vi "Translator.File.MatchStrings (Array).vi"(4 "sort? (T)":bool=TRUE, 5 "progressbar":refnum<vi>, 7 "group":string, 8 "error in":errorcluster, 9 "labels":string[](array[string]), 10 "default values":string[](array[string]), 11 "refnum in":T1) -> (0 "error out":errorcluster, 1 "#added":i32, 2 "values out":string[](array[string]), 3 "refnum out":T1)   [LabVIEW 2016]
uses:
  <vilib>/Utility/config.llb/Config Data RefNum.ctl
  <vilib>/Utility/config.llb/Write Key (String).vi
  <vilib>/Utility/config.llb/Read Key (String).vi
  <vilib>/Utility/config.llb/NI_LVConfig.lvlib
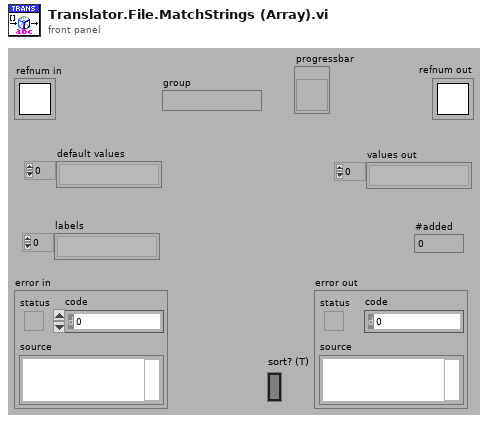
[diagram p1: front panel]
types:
  T1 = typedef "NI_LVConfig.lvlib/Config Data RefNum.ctl" = refnum<k1>
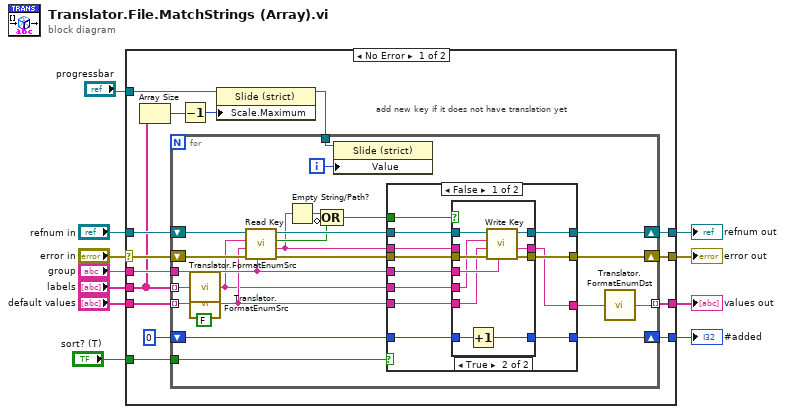
[diagram p0: block diagram]
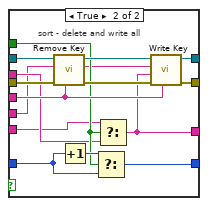
[diagram p3: hidden frame]
diagram:
  n1 = case shown="No Error" "error in" {
    selector: "error in" -> [w19 w91]
    tunnel: "refnum in" -> [w18 w92]
    tunnel: [w25 _] -> w10
    tunnel: [w24 w92] -> w9
    tunnel: [w23 w91] -> w8
    tunnel: [w22 w90] -> w7
    tunnel: "group" -> [w21 _]
    tunnel: "labels" -> [w15 _]
    tunnel: "default values" -> [w20 w90]
    tunnel: "progressbar" -> [w14 _]
    tunnel: "sort? (T)" -> [w12 _]
    frame No Error {
      # "add new key if it does not have translation yet"
      n2 = Array Size(array=w15) -> (size(s)=w17:i32)
      n3 = Decrement(x=w17) -> (x-1=w16:i32)
      n4 = property on="Property Node" class="Slide (strict)"(reference=w14, "Scale.Maximum"=w16) -> (reference out=w13:refnum<vi>)  [unwired: 1 in, 1 out]
      n5 = for {
        tunnel: w21 -> [w43]
        tunnel: w15 -> [w42] mode=indexing
        shift-right: [w46] -> w23
        shift-left: w19 -> [w49]
        shift-right: [w44] -> w24
        shift-left: w18 -> [w48]
        tunnel: [w28] -> w22 mode=indexing
        shift-right: [w34] -> w25
        shift-left: 0 -> [w35]
        tunnel: w20 -> [w41] mode=indexing
        tunnel: w13 -> [w32]
        tunnel: w12 -> [w29]
        i -> [w30]
        n6 = call "Translator.FormatEnumSrc.vi"("text in"=w42) -> ("text out"=w31:string)  [unwired: 1 in]
        n7 = call "Translator.FormatEnumSrc.vi"("text in"=w41, "quotas?(T)"=FALSE) -> ("text out"=w40:string)
        n8 = call-poly <vilib>:"Read Key.vi"("section"=w43, "error in (no error)"=w49, "default value"=w40, "key"=w31, "refnum"=w48) -> ("error out"=w47:errorcluster, "value"=w36:string, "found?"=w37:bool, "refnum out"=w45:T1)  [unwired: 3 in]
        n9 = Empty String/Path?(string/path=w36) -> (empty?=w39:bool)
        n10 = Compound Arithmetic op=OR(w39, invert w37) -> (w38:bool)
        n11 = property on="Property Node" class="Slide (strict)"(reference=w32, "Value"=w30) -> ()  [unwired: 1 in, 2 out]
        n12 = case shown="False" w29 {
          tunnel: w47 -> [w61 w89]
          tunnel: [w60 w84] -> w46
          tunnel: w45 -> [w59 w88]
          tunnel: [w58 w86] -> w44
          tunnel: w43 -> [w57 w83]
          tunnel: w40 -> [w56 w77]
          tunnel: w38 -> [w55 w79]
          tunnel: w36 -> [w54 w78]
          tunnel: w35 -> [w53 w82]
          tunnel: [w52 w80] -> w34
          tunnel: w31 -> [w51 w75]
          tunnel: [w50 w76] -> w27
          frame False {
            n13 = case shown="True" w55 {
              tunnel: w61 -> [w64 w74]
              tunnel: [w64 w73] -> w60
              tunnel: w59 -> [w65 w72]
              tunnel: [w65 w71] -> w58
              tunnel: w57 -> [_ w70]
              tunnel: w56 -> [_ w66]
              tunnel: w54 -> [w63 _]
              tunnel: w51 -> [_ w69]
              tunnel: [w63 w66] -> w50
              tunnel: w53 -> [w62 w68]
              tunnel: [w62 w67] -> w52
              frame False {
              }
              frame True {
                n14 = Increment(x=w68) -> (x+1=w67:i32)
                n15 = call-poly <vilib>:"Write Key.vi"("section"=w70, "error in (no error)"=w74, "value"=w66, "key"=w69, "refnum"=w72) -> ("error out"=w73:errorcluster, "refnum out"=w71:T1)  [unwired: 4 in, 1 out]
              }
            }
          }
          frame True {
            # "sort - delete and write all"
            n16 = call <vilib>:"Remove Key.vi"("section"=w83, "error in (no error)"=w89, "key"=w75, "refnum"=w88) -> ("error out"=w85:errorcluster, "refnum out"=w87:T1)  [unwired: 5 in, 1 out]
            n17 = Increment(x=w82) -> (x+1=w81:i32)
            n18 = Select(t=w81, s=w79, f=w82) -> (s? t:f=w80:i32)
            n19 = Select(t=w77, s=w79, f=w78) -> (s? t:f=w76:string)
            n20 = call-poly <vilib>:"Write Key.vi"("section"=w83, "error in (no error)"=w85, "value"=w76, "key"=w75, "refnum"=w87) -> ("error out"=w84:errorcluster, "refnum out"=w86:T1)  [unwired: 4 in, 1 out]
          }
        }
        n21 = call "Translator.FormatEnumDst.vi"("text in"=w27) -> ("text out"=w28:string)
      }
    }
    frame Error {
    }
  }
  "#added" <- w10
  "refnum out" <- w9
  "error out" <- w8
  "values out" <- w7
